vi "Unified Actor Lifetime.vi"(7 "Actor in":refnum<class "Actor.lvclass">) -> (2 "Unified Actor Lifetime":T1)   [LabVIEW 2020, in "jettl.lvlib" / "Read Base Actor.lvlib"]
uses:
  Read Base Actor.lvlib
  Actor/Actor.lvclass
  Unified Actor Lifetime.ctl
  jettl.lvlib
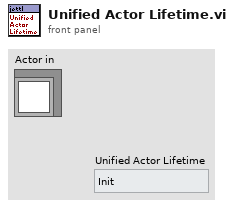
[diagram p1: front panel]
types:
  T1 = typedef "jettl.lvlib/Unified Actor Lifetime.ctl" = enum16{"Init", "Spawn", "Setup", "Teardown Before Running", "Running", "Stop Called", "Stopping With Children", "Stopping Without Children", "Teardown After Running", "Stopped"}
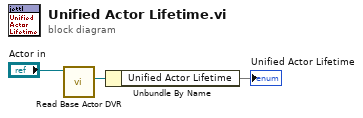
[diagram p0: block diagram]
diagram:
  n1 = call-dynamic "Read Base Actor DVR.vi"("Actor in"="Actor in") -> ("Base Actor DVR"=w2:refnum<data-value>)  [unwired: 10 in]
  n2 = Unbundle By Name(w2) -> ("Unified Actor Lifetime"=→"Unified Actor Lifetime")
